vi "Return Message.vi"(8 "error in (no error)":errorcluster, 9 "Connection ID":string, 10 "Message To Return":refnum<class "IPacket.lvclass">, 11 "IMessageReturnPolicy in":refnum<class "IMessageReturnPolicy.lvclass">) -> (0 "error out":errorcluster)   [LabVIEW 2019, in "MessagingInterfaces.lvlib" / "IMessageReturnPolicy.lvclass"]
uses:
  <vilib>/gpm_packages/@cs/Network-interface/Source/MessagingInterfaces/IMessageReturnPolicy/IMessageReturnPolicy.lvclass
  <vilib>/gpm_packages/@cs/Network-interface/Source/MessagingInterfaces/IPacket/IPacket.lvclass
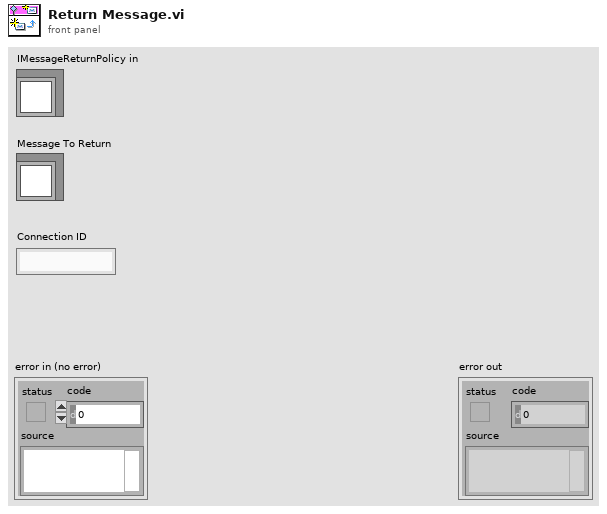
[diagram p1: front panel]
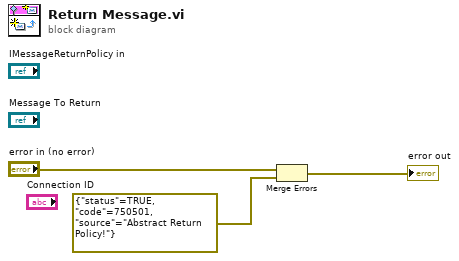
[diagram p0: block diagram]
diagram:
  n1 = Merge Errors("error in (no error)", errorcluster {"status"=TRUE, "code"=750501, "source"="Abstract Return Policy!"} ("error in")) -> (→"error out":errorcluster)
